vi "Start.vi"(5 "Autoshutdown? (T)":bool=TRUE, 7 "StartupParams":variant, 8 "error in (no error)":errorcluster, 11 "JQMHCore in":refnum<class "Module.lvclass">) -> (0 "error out":errorcluster, 1 "StartupHandshake out":refnum<class "ModuleStartup.lvclass">, 3 "JQMHCore out":refnum<class "Module.lvclass">)   [LabVIEW 2024, in "Module.lvclass"]
uses:
  Module.lvclass
  Startup/ModuleStartup.lvclass
  Module.lvclass/Module.ctl
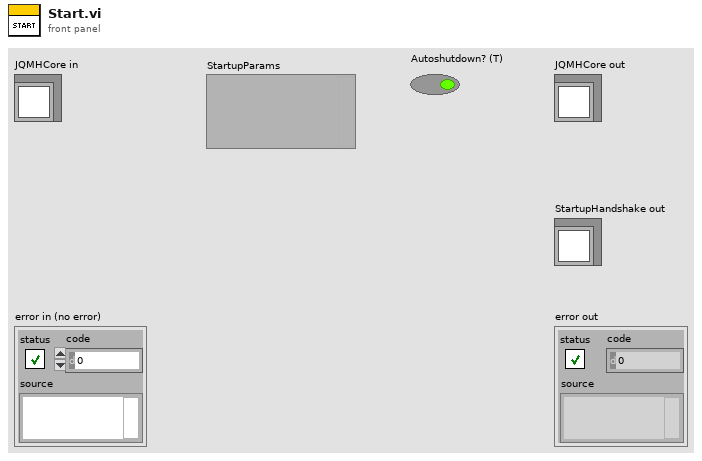
[diagram p1: front panel]
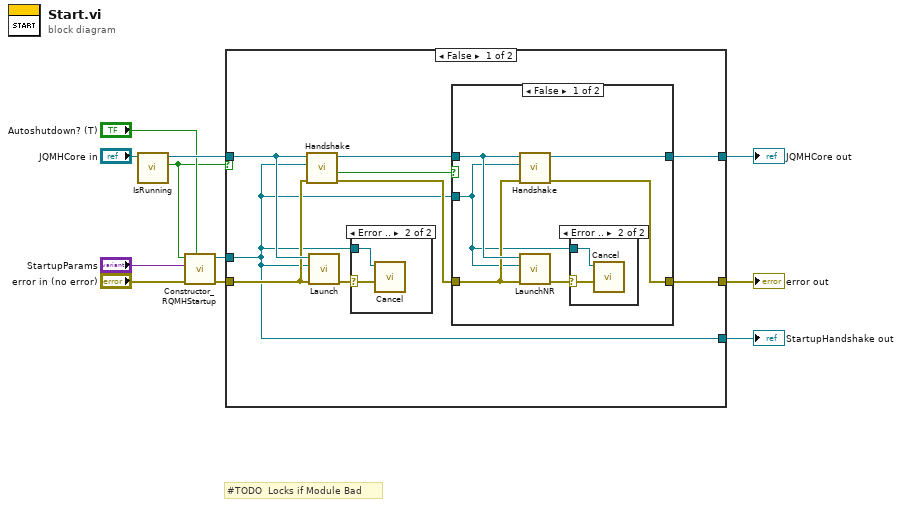
[diagram p0: block diagram]
diagram:
  # "#TODO  Locks if Module Bad"
  n1 = call "IsRunning.vi"("JQMHModule in"="JQMHCore in") -> ("Is Running?"=w3:bool, "JQMHModule out"=w6:refnum<class "Module.lvclass">)  [unwired: 9 in]
  n2 = call "Constructor_RQMHStartup.vi"("Autoshutdown? (T)"="Autoshutdown? (T)", "error in (no error)"="error in (no error)", "StartupParams"="StartupParams", "Already Running?"=w3) -> ("error out"=w5:errorcluster, "JQMHStartup out"=w2:refnum<class "ModuleStartup.lvclass">)  [unwired: 6 in]
  n3 = case shown="False" w3 {
    tunnel: [w20 w34] -> w10
    tunnel: [w19 w35] -> w9
    tunnel: w6 -> [w18 w35]
    tunnel: w5 -> [w14 w34]
    tunnel: w2 -> [w12 w33]
    tunnel: [w12 w33] -> w1
    frame False {
      n4 = call "Handshake.vi"("error in (no error)"=w14, "JQMHStartup in"=w12, "JQMHModule in"=w18) -> ("error out"=w13:errorcluster, "HandshakeComplete?"=w16:bool, "JQMHModule out"=w17:refnum<class "Module.lvclass">)  [unwired: 6 in]
      n5 = call "Launch.vi"("error in (no error)"=w14, "JQMHStartup"=w12, "JQMHCore in"=w18) -> ("error out"=w15:errorcluster)  [unwired: 8 in]
      n6 = case shown="Error .." w15 {
        selector: w15 -> [_ w22]
        tunnel: w12 -> [_ w21]
        frame No Error {
        }
        frame Error {
          n7 = call "Cancel.vi"("CancellationReason"=w22, "JQMHStartup in"=w21) -> ()  [unwired: 9 in, 1 out]
        }
      }
      n8 = case shown="False" w16 {
        tunnel: w13 -> [w25 w31]
        tunnel: w12 -> [w23 _]
        tunnel: w17 -> [w28 w32]
        tunnel: [w26 w31] -> w20
        tunnel: [w27 w32] -> w19
        frame False {
          n9 = call "Handshake.vi"("error in (no error)"=w25, "JQMHStartup in"=w23, "JQMHModule in"=w28) -> ("error out"=w26:errorcluster, "JQMHModule out"=w27:refnum<class "Module.lvclass">)  [unwired: 6 in, 1 out]
          n10 = call "LaunchNR.vi"("error in (no error)"=w25, "JQMHStartup"=w23, "JQMHCore in"=w28) -> ("error out"=w24:errorcluster)  [unwired: 8 in]
          n11 = case shown="Error .." w24 {
            selector: w24 -> [_ w30]
            tunnel: w23 -> [_ w29]
            frame No Error {
            }
            frame Error {
              n12 = call "Cancel.vi"("CancellationReason"=w30, "JQMHStartup in"=w29) -> ()  [unwired: 9 in, 1 out]
            }
          }
        }
        frame True {
        }
      }
    }
    frame True {
    }
  }
  "error out" <- w10
  "JQMHCore out" <- w9
  "StartupHandshake out" <- w1
